vi "Force Quit.VI"   [LabVIEW 2019]
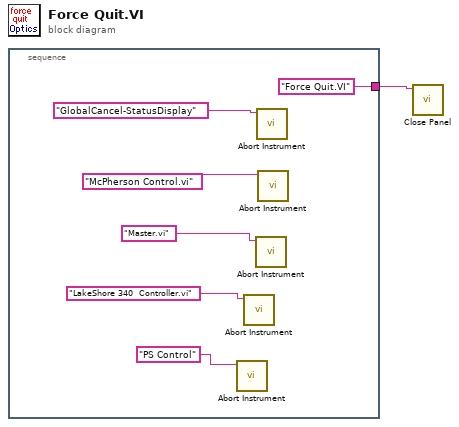
[diagram p0: block diagram]
diagram:
  n1 = stacked-sequence {
    tunnel: ["Force Quit.VI" ("name or relative path")] -> w1
    frame #0 {
      n2 = call <vilib>:"Abort Instrument.vi"("VI name"="PS Control" ("name or relative path")) -> ()  [unwired: 10 in, 1 out]
      n3 = call <vilib>:"Abort Instrument.vi"("VI name"="LakeShore 340  Controller.vi" ("name or relative path")) -> ()  [unwired: 10 in, 1 out]
      n4 = call <vilib>:"Abort Instrument.vi"("VI name"="Master.vi" ("name or relative path")) -> ()  [unwired: 10 in, 1 out]
      n5 = call <vilib>:"Abort Instrument.vi"("VI name"="GlobalCancel-StatusDisplay" ("name or relative path")) -> ()  [unwired: 10 in, 1 out]
      n6 = call <vilib>:"Abort Instrument.vi"("VI name"="McPherson Control.vi" ("name or relative path")) -> ()  [unwired: 10 in, 1 out]
    }
  }
  n7 = call <vilib>:"Close Panel.vi"("VI name"=w1) -> ()  [unwired: 10 in, 1 out]
